vi "Reset Timer OFF Cycle.vi"(8 "error in (no error)":errorcluster, 10 "Main_Burner_Flag_Out":u8, 11 "Timer in":refnum<queue>) -> (0 "error out":errorcluster)   [LabVIEW 2023]
uses:
  Message Queue/Message Cluster.ctl
  controls/Burner Duty Cycle.ctl
  Message Queue/Enqueue Message (Single).vi
  Message Queue/Message Queue.lvlib
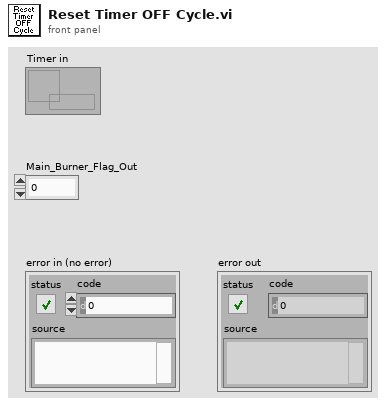
[diagram p1: front panel]
types:
  T1 = typedef "Burner Duty Cycle.ctl" = cluster{"Burner ON Time (Seconds)":dbl, "Burner OFF Time (Seconds)":dbl, "Main Burner Flag":bool, "Burner Power Mode":u8}
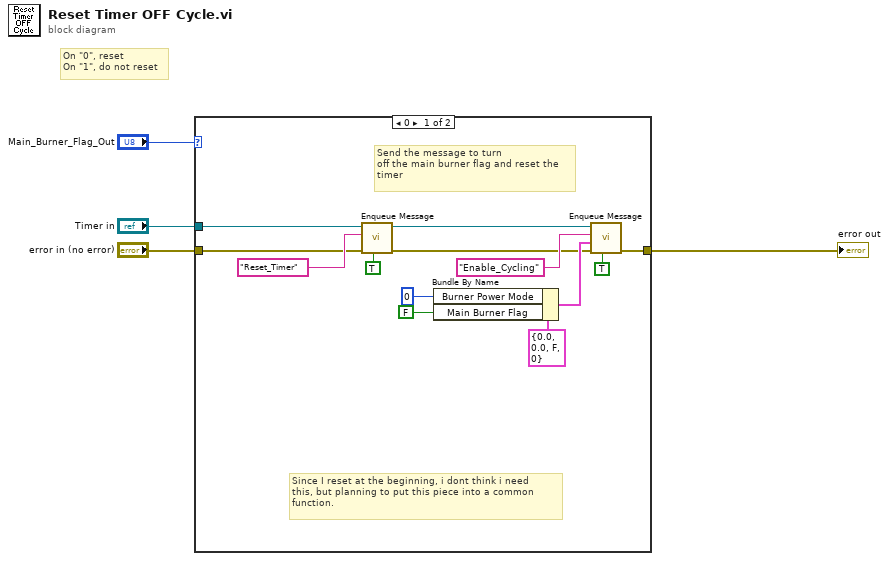
[diagram p0: block diagram]
diagram:
  # "On \"0\", reset\nOn \"1\", do not reset"
  n1 = case shown="0" "Main_Burner_Flag_Out" {
    tunnel: "error in (no error)" -> [w9 w18]
    tunnel: [w15 w18] -> w2
    tunnel: "Timer in" -> [w7 _]
    frame 0 {
      # "Since I reset at the beginning, i dont think i need\nthis, but planning to put this piece into a common \nfunction."
      # "Send the message to turn\noff the main burner flag and reset the\ntimer"
      n2 = call-poly "Enqueue Message.vi"("Priority Message? (F)"=TRUE, "error in (no error)"=w9, "Message"="Reset_Timer", "Message Queue"=w7) -> ("error out"=w8:errorcluster, "dup Message Queue"=w6:refnum<queue>)  [unwired: 6 in]
      n3 = Bundle By Name(cluster=T1 {"Burner ON Time (Seconds)"=0.0, "Burner OFF Time (Seconds)"=0.0, "Main Burner Flag"=FALSE, "Burner Power Mode"=0} ("Duty Cycle"), "Burner Power Mode"=u8 0, "Main Burner Flag"=FALSE) -> (w13:T1)
      n4 = call-poly "Enqueue Message.vi"("Priority Message? (F)"=TRUE, "error in (no error)"=w8, "Message Data"=w13, "Message"="Enable_Cycling", "Message Queue"=w6) -> ("error out"=w15:errorcluster)  [unwired: 5 in, 1 out]
    }
    frame 1, Default {
      # "If the flag is enabled, do nothing."
    }
  }
  "error out" <- w2
